vi "chaos crest push.vi"(10 "cu_uid":u32, 11 "handleConnection":u32) -> (3 "nok":i32)   [LabVIEW 2014, in "libcommon-crest.lvlib"]
doc: "int chaos_crest_push(chaos_crest_handle_t h,uint32_t cu_uid);"
uses:
  libcommon-crest.lvlib
  chaos-i686-dynamic-release/lib/libcommon-crest.so
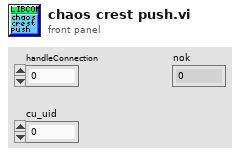
[diagram p1: front panel]
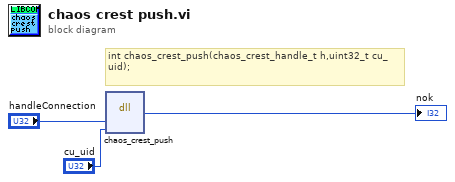
[diagram p0: block diagram]
diagram:
  # "int chaos_crest_push(chaos_crest_handle_t h,uint32_t cu_uid);"
  n1 = dll-call lib="home/chaos/chaos_bundle/chaos-i686-dynamic-release/lib/libcommon-crest.*" fn="chaos_crest_push"("handleConnection"="handleConnection", "cu_uid"="cu_uid") -> (→"nok":i32)  [unwired: 5 in, 2 out]
